vi "Get-pane.vi"(8 "error in (no error)":errorcluster, 10 "Pane":T2, 11 "Panes in":T5) -> (0 "error out":errorcluster, 1 "Index":i32, 2 "Pane":T1, 3 "Panes out":T5)   [LabVIEW 2013, in "PaneToggle.lvlib" / "Panes.lvclass"]
uses:
  Panes.lvclass
  Object-reference.ctl
  Pane-names.ctl
  Pane-settings.ctl
  Splitter-settings.ctl
  Splitter-names.ctl
  Panes.lvclass/Panes.ctl
  Read-Panes.vi
  <vilib>/Utility/error.llb/Error Cluster From Error Code.vi
  <vilib>/ErrorRing/Error Ring.xnode
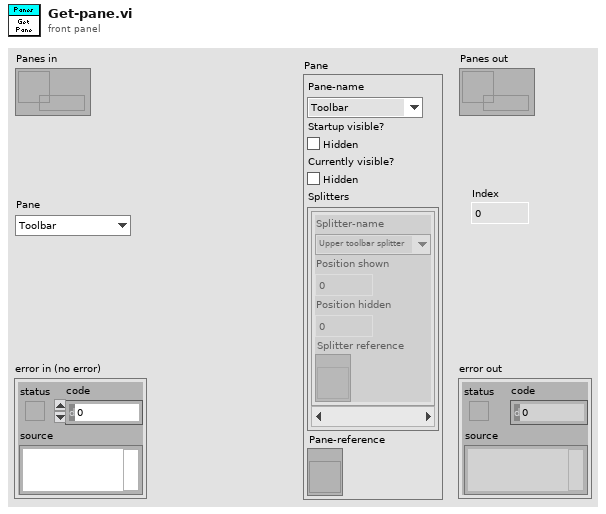
[diagram p1: front panel]
types:
  T1 = typedef "PaneToggle.lvlib/Panes.lvclass/Pane-settings.ctl" = cluster{"Pane-name":T2, "Startup visible?":bool, "Currently visible?":bool, "Splitters":T3[], "Pane-reference":refnum<vi>}
  T2 = typedef "PaneToggle.lvlib/Panes.lvclass/Pane-names.ctl" = enum16{"Toolbar", "Help bar", "Toolbar lower border", "Main panel", "Status bar upper border", "General state bar", "Information bar"}
  T3 = typedef "PaneToggle.lvlib/Panes.lvclass/Splitter-settings.ctl" = cluster{"Splitter-name":T4, "Position shown":i32, "Position hidden":i32, "Splitter reference":refnum<vi>}
  T4 = typedef "PaneToggle.lvlib/Panes.lvclass/Splitter-names.ctl" = enum16{"Upper toolbar splitter", "Help bar splitter", "Lower toolbar splitter", "Upper status bar splitter", "Lower status bar splitter", "Left status bar splitter"}
  T5 = typedef "PaneToggle.lvlib/Panes.lvclass/Object-reference.ctl" = refnum<data-value>
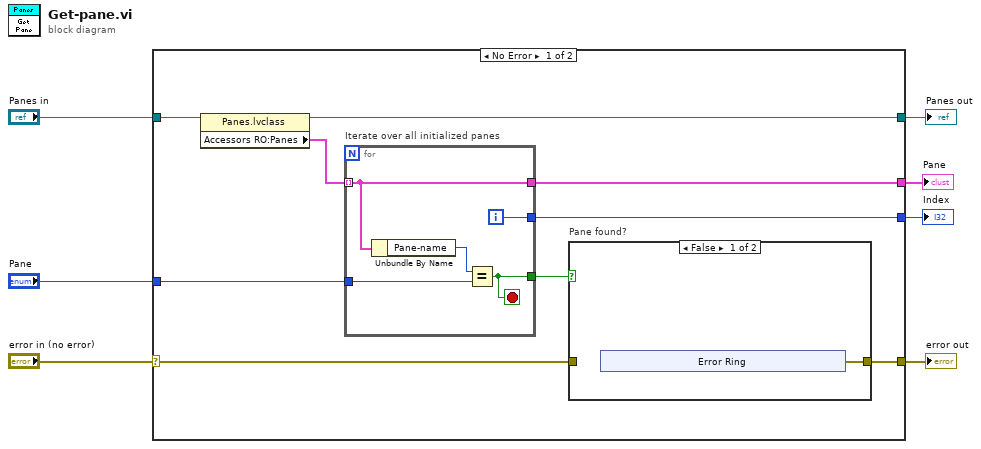
[diagram p0: block diagram]
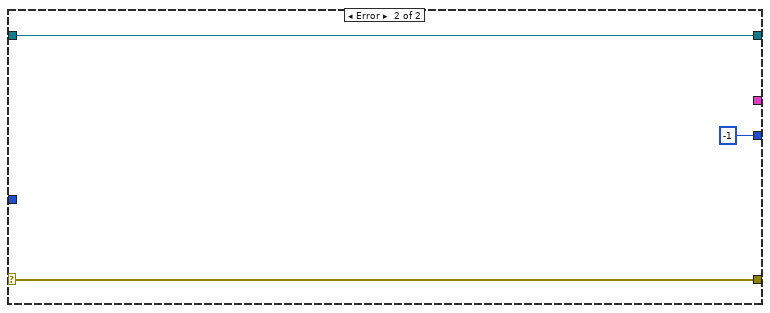
[diagram p3: hidden frame]
diagram:
  n1 = case shown="No Error" "error in (no error)" {
    selector: "error in (no error)" -> [w12 w29]
    tunnel: [w11 w29] -> w6
    tunnel: [w13 w30] -> w4
    tunnel: "Panes in" -> [w16 w30]
    tunnel: "Pane" -> [w14 _]
    tunnel: [w9 _] -> w2
    tunnel: [w8 -1] -> w1
    frame No Error {
      n2 = property class="Panes.lvclass"(reference=w16) -> (reference out=w13:T5, "Accessors RO:Panes"=w15:T1[])  [unwired: 1 in, 1 out]
      n3 = for "Iterate over all initialized panes" {
        tunnel: w15 -> [w24] mode=indexing
        tunnel: w14 -> [w27]
        tunnel: [w25] -> w10
        tunnel: [w24] -> w9
        tunnel: [w23] -> w8
        i -> [w23]
        stop <- w25 stop-if-true
        n4 = Unbundle By Name(w24) -> ("Pane-name"=w26:T2)
        n5 = Equal?(x=w26, y=w27) -> (x = y?=w25:bool)
      }
      n6 = case "Pane found?" shown="False" w10 {
        tunnel: w12 -> [_ w22]
        tunnel: [w17 w22] -> w11
        frame False {
          n7 = xnode "Error Ring"() -> ("error out"=w17:errorcluster)
        }
        frame True {
        }
      }
    }
    frame Error {
    }
  }
  "error out" <- w6
  "Panes out" <- w4
  "Pane" <- w2
  "Index" <- w1
